vi "ZNB initialization.vi"(8 "error in (no error)":errorcluster, 9 "Output port":i32, 10 "Input port":i32, 11 "VISA resource name":refnum<visa-resource-name>) -> (0 "error out":errorcluster)   [LabVIEW 2015]
uses:
  <instrlib>/Rohde&Schwarz Vector Network Analyzer/Rohde&Schwarz Vector Network Analyzer.lvlib
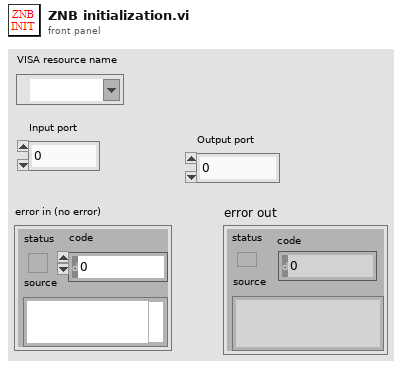
[diagram p1: front panel]
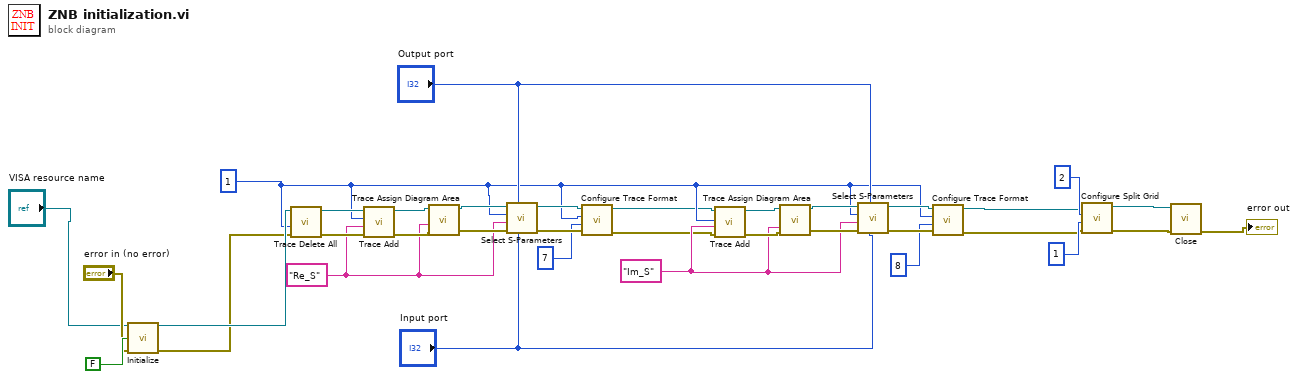
[diagram p0: block diagram]
diagram:
  w17 = "Im_S"
  w22 = "Re_S"
  w11 = 1
  n1 = call <instrlib>:"Initialize.vi"("VISA resource name"="VISA resource name", "Reset (T: Reset)"=FALSE, "error in (no error)"="error in (no error)") -> ("VISA resource name out"=w14:refnum<visa-resource-name>, "error out"=w12:errorcluster)  [unwired: 11 in]
  n2 = call <instrlib>:"Trace Delete All.vi"("error in (no error)"=w12, "Channel (1)"=w11, "VISA resource name"=w14) -> ("error out"=w34:errorcluster, "VISA resource name out"=w35:refnum<visa-resource-name>)  [unwired: 7 in]
  n3 = call <instrlib>:"Trace Add.vi"("error in (no error)"=w34, "Trace Name (\"Trc1\")"=w22, "Channel (1)"=w11, "VISA resource name"=w35) -> ("error out"=w24:errorcluster, "VISA resource name out"=w23:refnum<visa-resource-name>)  [unwired: 6 in]
  n4 = call <instrlib>:"Trace Assign Diagram Area.vi"("error in (no error)"=w24, "Trace Name (\"Ch1Trc1\")"=w22, "VISA resource name"=w23) -> ("error out"=w32:errorcluster, "VISA resource name out"=w33:refnum<visa-resource-name>)  [unwired: 7 in]
  n5 = call <instrlib>:"Select S-Parameters.vi"("In Port (1)"="Input port", "Out Port (1)"="Output port", "error in (no error)"=w32, "Trace Name (\"Trc1\")"=w22, "Channel (1)"=w11, "VISA resource name"=w33) -> ("error out"=w30:errorcluster, "VISA resource name out"=w31:refnum<visa-resource-name>)  [unwired: 4 in]
  n6 = call <instrlib>:"Configure Trace Format.vi"("error in (no error)"=w30, "Format (dB Mag)"=7, "Channel (1)"=w11, "VISA resource name"=w31) -> ("error out"=w5:errorcluster, "VISA resource name out"=w6:refnum<visa-resource-name>)  [unwired: 6 in]
  n7 = call <instrlib>:"Trace Add.vi"("error in (no error)"=w5, "Trace Name (\"Trc1\")"=w17, "Channel (1)"=w11, "VISA resource name"=w6) -> ("error out"=w20:errorcluster, "VISA resource name out"=w21:refnum<visa-resource-name>)  [unwired: 6 in]
  n8 = call <instrlib>:"Trace Assign Diagram Area.vi"("error in (no error)"=w20, "Trace Name (\"Ch1Trc1\")"=w17, "VISA resource name"=w21) -> ("error out"=w27:errorcluster, "VISA resource name out"=w28:refnum<visa-resource-name>)  [unwired: 7 in]
  n9 = call <instrlib>:"Select S-Parameters.vi"("In Port (1)"="Input port", "Out Port (1)"="Output port", "error in (no error)"=w27, "Trace Name (\"Trc1\")"=w17, "Channel (1)"=w11, "VISA resource name"=w28) -> ("error out"=w25:errorcluster, "VISA resource name out"=w26:refnum<visa-resource-name>)  [unwired: 4 in]
  n10 = call <instrlib>:"Configure Trace Format.vi"("error in (no error)"=w25, "Format (dB Mag)"=8, "Channel (1)"=w11, "VISA resource name"=w26) -> ("error out"=w7:errorcluster, "VISA resource name out"=w8:refnum<visa-resource-name>)  [unwired: 6 in]
  n11 = call <instrlib>:"Configure Split Grid.vi"("error in (no error)"=w7, "Columns (1)"=1, "Rows (1)"=2, "VISA resource name"=w8) -> ("error out"=w4:errorcluster, "VISA resource name out"=w3:refnum<visa-resource-name>)  [unwired: 6 in]
  n12 = call <instrlib>:"Close.vi"("error in (no error)"=w4, "VISA resource name"=w3) -> ("error out"=→"error out":errorcluster)  [unwired: 9 in]
